vi "PupilAnalysis.vi"() -> ()   [LabVIEW 2013]
uses:
  <vilib>/picture/picture.llb/imagedata.ctl
  <vilib>/Analysis/baseanly.llb/Mean (DBL).vi
  <vilib>/Analysis/2dsp.llb/1D Convolution (DBL).vi
  <vilib>/Analysis/2dsp.llb/Decimate (single shot, DBL).vi
  <vilib>/Analysis/1siggen.llb/General Aperiodic Triangle.vi
  <vilib>/measure/maresamp.llb/Resample N Waveforms (single shot).vi
  <vilib>/measure/macond.llb/IIR Filter for N Chan.vi
  <vilib>/imath/engines/lvmath2/RunTimeEngine/ErrorHandling/NIMS_Finalize Error.vi
  <vilib>/imath/engines/lvmath2/RunTimeEngine/BuiltInFunctions/length/NIMS_length(GV).vi
  <instcachedir>/0/NIMS_length(GV)_08A3D13377FD4E4B96F5795FBF3698FA.lvgen/NIMS_length(GV)_08A3D13377FD4E4B96F5795FBF3698FA_000.vi
  <vilib>/imath/engines/lvmath2/RunTimeEngine/BuiltInFunctions/zeros/NIMS_V=zeros(I32,I32).vi
  <vilib>/imathl/engines/lvmath/Functions/Error Handling/Create Error.vi
  <vilib>/imath/engines/lvmath/Plug In/_Char/NIMS_CH_String to Character Array.vi
  <vilib>/imath/engines/lvmath2/RunTimeEngine/VariableToken/NIMS_VariableToken_CondDefined.vi
  <instcachedir>/0/NIMS_VariableToken_CondDefined_9DC5CEC47F8146B087FA2781C705B229.lvgen/NIMS_VariableToken_CondDefined_9DC5CEC47F8146B087FA2781C705B229_003.vi
  <vilib>/imath/engines/lvmath/Functions/Error Handling/MergeErrorsWrapper.vi
  <vilib>/imath/engines/lvmath2/RunTimeEngine/NodeEndStatement/NIMS_NodeEndStatement_Output.vi
  <instcachedir>/0/NIMS_NodeEndStatement_Output_53EC0D466D134D7ABD903AC30B43404B.lvgen/NIMS_NodeEndStatement_Output_53EC0D466D134D7ABD903AC30B43404B_005.vi
  <instcachedir>/0/NIMS_NodeEndStatement_Output_53EC0D466D134D7ABD903AC30B43404B.lvgen/NIMS_NodeEndStatement_Output_53EC0D466D134D7ABD903AC30B43404B_004.vi
  <vilib>/imath/engines/lvmath2/RunTimeEngine/RangeToken/NIMS_Range_R2 - Integer.vi
  <instcachedir>/0/NIMS_Range_R2 - Integer_C51C130E5EA5464EA148B28CDAB9615A.lvgen/NIMS_Range_R2 - Integer_C51C130E5EA5464EA148B28CDAB9615A_000.vi
  <vilib>/imath/engines/lvmath2/RunTimeEngine/CommandStatement/MC_CommandStatement_break.vi
  <vilib>/imath/engines/lvmath2/RunTimeEngine/IndexRead/NIMS V(S).vi
  <instcachedir>/0/NIMS V(S)_0488751826AF41519A22953C041130DC.lvgen/NIMS V(S)_0488751826AF41519A22953C041130DC_000.vi
  <vilib>/imath/engines/lvmath2/RunTimeEngine/ErrorHandling/NIMS_Create Error From Enums.vi
  <vilib>/imath/engines/lvmath2/RunTimeEngine/IndexReplace/NIMS V(S)=S.vi
  <instcachedir>/0/NIMS V(S)=S_66A18068148B4981A312229A93EA5C06.lvgen/NIMS V(S)=S_66A18068148B4981A312229A93EA5C06_003.vi
  <vilib>/imath/engines/lvmath2/RunTimeEngine/RangeToken/NIMS_Range.vi
  <instcachedir>/0/NIMS_Range_7481B155BEE341ECA0F59DDB444E2C09.lvgen/NIMS_Range_7481B155BEE341ECA0F59DDB444E2C09_000.vi
  <vilib>/imath/engines/lvmath2/RunTimeSupport/NIMS_Error if Not Equal.vi
  <instcachedir>/0/NIMS_Error if Not Equal_902F5D2649E64F5087A1EF57C55C58AB.lvgen/NIMS_Error if Not Equal_902F5D2649E64F5087A1EF57C55C58AB_001.vi
  <vilib>/imath/engines/lvmath2/RunTimeEngine/IndexRead/NIMS V(V).vi
  <instcachedir>/0/NIMS V(V)_298D9CB7BFEB42B8BC8D9C3C28AE8C70.lvgen/NIMS V(V)_298D9CB7BFEB42B8BC8D9C3C28AE8C70_000.vi
  <vilib>/imath/engines/lvmath2/RunTimeEngine/BuiltInFunctions/max/1 input/NIMS_max(RV).vi
  <instcachedir>/0/NIMS_max(RV)_237633DB1D604D5BA7001287DF3C7957.lvgen/NIMS_max(RV)_237633DB1D604D5BA7001287DF3C7957_002.vi
  <instcachedir>/0/NIMS V(S)_0488751826AF41519A22953C041130DC.lvgen/NIMS V(S)_0488751826AF41519A22953C041130DC_002.vi
  <vilib>/imath/engines/lvmath/Plug In/_Char/NIMS_CH_Character RV to String.vi
  <vilib>/imath/engines/lvmath2/RunTimeSupport/NIMS_String to Enum.vi
  <vilib>/imath/engines/lvmath2/RunTimeEngine/BuiltInFunctions/interpolate1d/NIMS_interpolate1d(RV,RV,RV,Str).vi
  <instcachedir>/0/NIMS_Error if Not Equal_902F5D2649E64F5087A1EF57C55C58AB.lvgen/NIMS_Error if Not Equal_902F5D2649E64F5087A1EF57C55C58AB_000.vi
  <instcachedir>/0/NIMS V(S)=S_66A18068148B4981A312229A93EA5C06.lvgen/NIMS V(S)=S_66A18068148B4981A312229A93EA5C06_000.vi
  <vilib>/imath/engines/lvmath2/RunTimeEngine/VariableToken/NIMS_VariableToken_CondDefinedDefinedByReplace.vi
  <instcachedir>/0/NIMS_VariableToken_CondDefinedDefinedByReplace_D162CFFC24174562A9FEA619A91E1A56.lvgen/NIMS_VariableToken_CondDefinedDefinedByReplace_D162CFFC24174562A9FEA619A91E1A56_002.vi
  <vilib>/Waveform/WDTFileIO.llb/ Write Waveforms to File (1D).vi
  <vilib>/Utility/file.llb/Read From Spreadsheet File (DBL).vi
  <vilib>/Utility/file.llb/Write To Spreadsheet File (DBL).vi
  <vilib>/Analysis/NI_AALBase.lvlib
  <vilib>/Analysis/NI_AALPro.lvlib
  <vilib>/measure/NI_MAPro.lvlib
  <vilib>/gmath/NI_Gmath.lvlib
panel:
  out "Tab Control":T1(tab)
  in  "Save Cleaned Data":bool
  in  "Apply New Settings":bool
  out "Cleaned Data":dynamicdata(graph)
  in  "New Sample Rate (Hz)":i32=25
  out "file information":string
  out "raw data":dbl[][](array[numeric])
  out "Unprocessed Data":waveform(dbl)[](graph)
  in  "Analyse Responses":bool
  in  "Rank":i32=3 min=1
  in  "Filter?":bool
  in  "Median Filter?":bool
  in  "max pupil width":dbl=0.4 format="%.2f"
  in  "min pupil width":dbl=0.1 format="%.2f"
  in  "min Aspect Ratio":dbl=0.7
  in  "Blink Window Length":dbl=5.0
  in  "Interpolation":u16(ring)=1 items=["Spline", "Linear"]
  in  "Resample Data":bool
  out "Sample Rate (Hz)":dbl format="%0.2f"
  in  "IIR filter specifications":T2={"Topology"=enum."Butterworth", "Type"=enum."Lowpass", "Order"=1, "Lower Fc"=10.0, "Upper Fc"=200.0, "PB Ripple"=1.0, "SB Attenuation"=60.0} {"PB Ripple" format="%0.2f"; "SB Attenuation" format="%0.2f"; "Lower Fc" format="%0.2p"; "Upper Fc" format="%0.2p"}
  out "Image onsets":string[](array[string])
  in  "Save Between Cursors":bool
  in  "Save Coefficients":bool
  out "Basis Set":dbl[][](graph)
  out "Event-related responses":dbl[][](graph)
  out "All Regressors":dbl[][](graph)
  out "Data and Fitted Response":dynamicdata(graph)
  in  "Timing Files":path[](array[path])
  in  "Number of Basis Functions":i32=15
  in  "Window Length (s)":dbl=10.0
  out "Coefficients":dbl[](array[numeric])
  in  "finished":bool
  in  "recalculate":bool
  in  "Save Response Data":bool
  in  "decimating factor":i32=1
  in  "Basis Set":u16(ring)=1 items=["Fourier", "Tents", "Blocks"]
  out "X * Y":dbl[](array[numeric])
  out "2D Picture":picture
  in  "next picture":bool
  out "image data":T3
  in  "Images Directory":path=path "E:/Documents/IAPS/bmp/800x600"
  in  "Objects Directory":path=path "E:/Documents/IAPS/objects"
  out "object file":path
  out "Image file":path
  out "Image Number":i32
  out "2D Picture 2":picture
  out "Fixations in ROIs":dbl[][](array[numeric])
  in  "Post-Picture Window Length":i32
  # "Data Cleaning"
  # "Pupil Dilation Analysis"
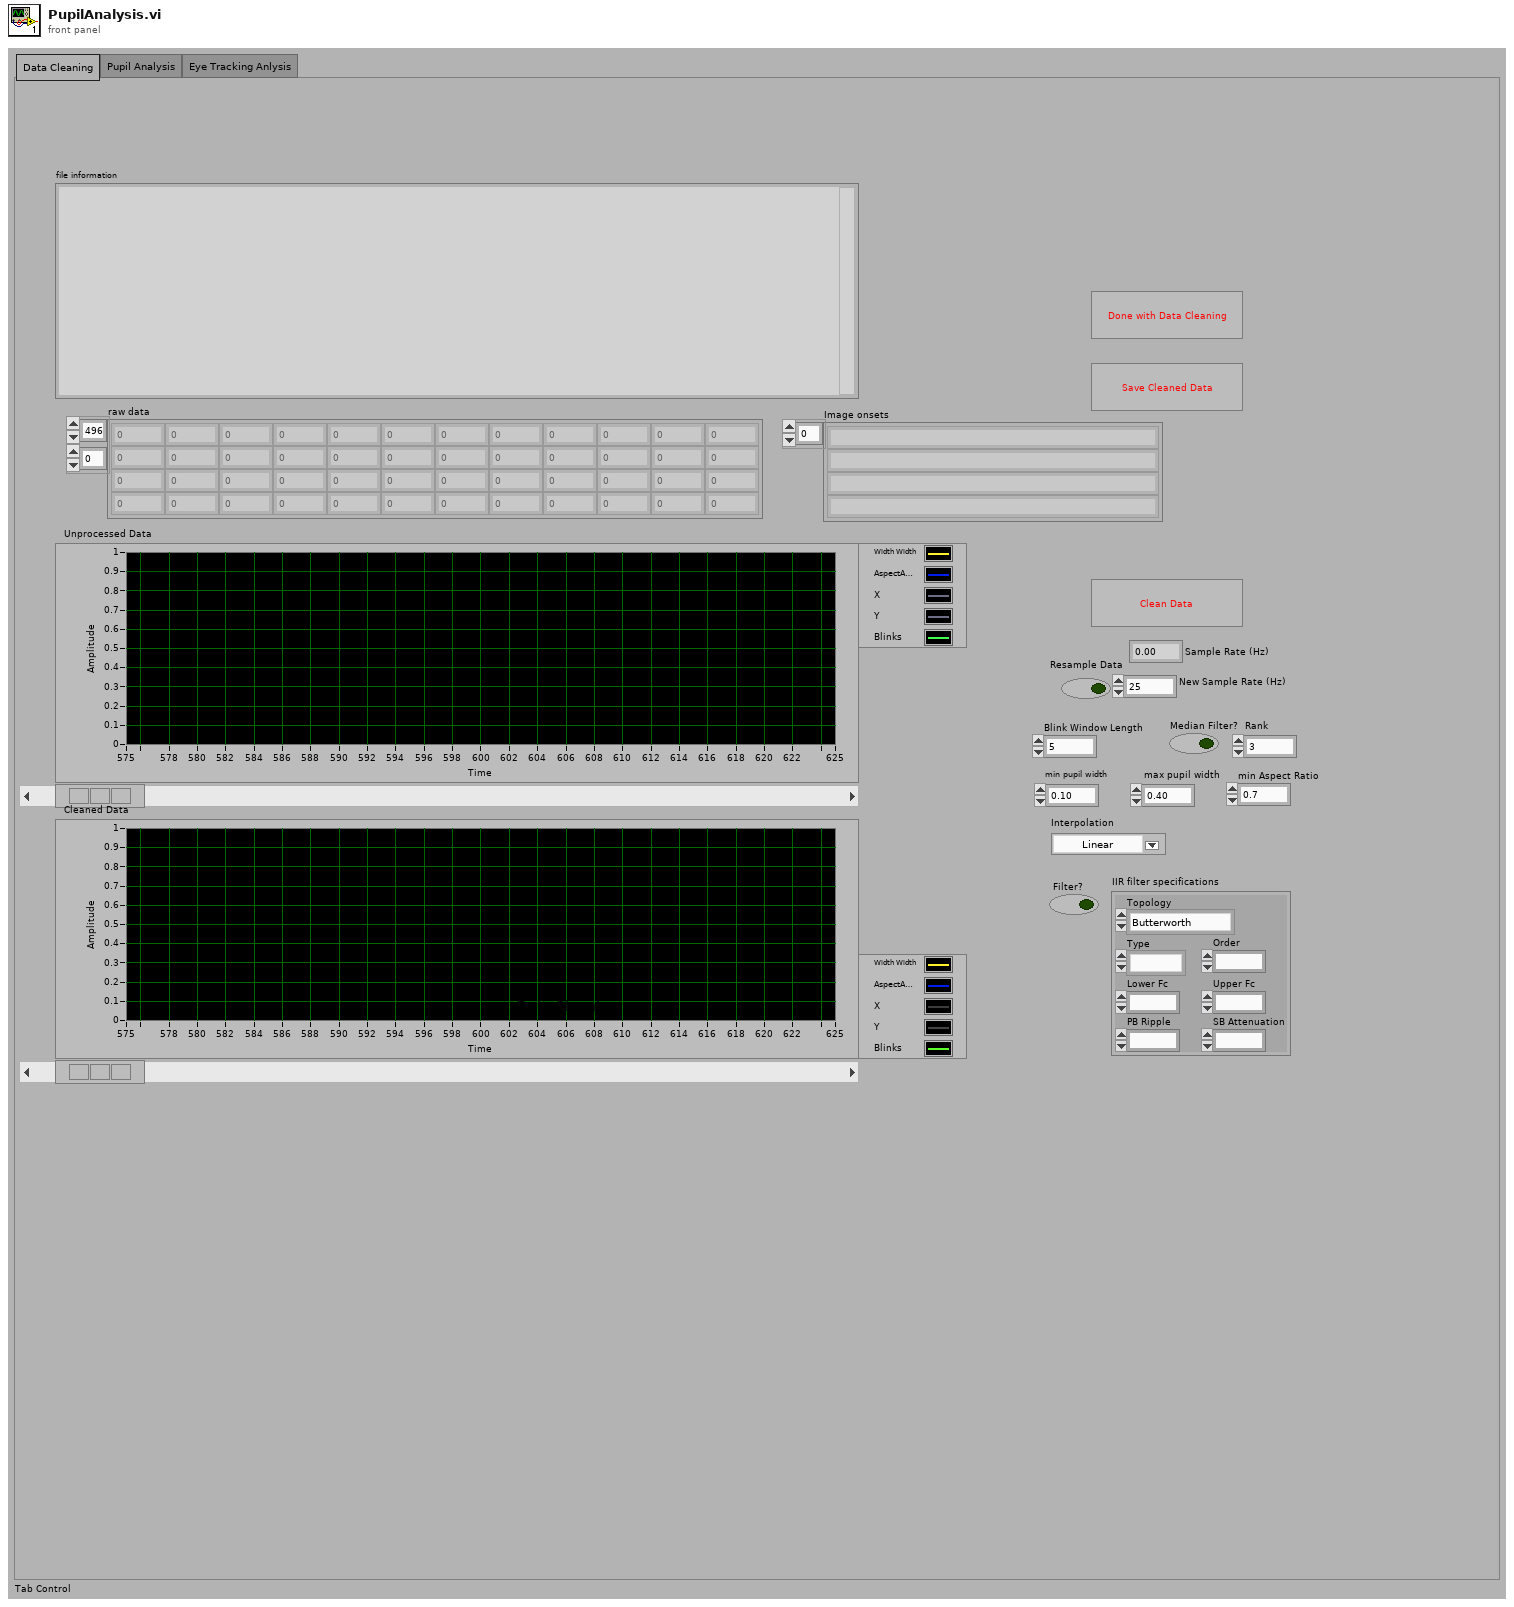
[diagram p1: front panel]
types:
  T1 = enum32{"Data Cleaning", "Pupil Analysis", "Eye Tracking Anlysis"}
  T2 = cluster{"Topology":enum16{"Off", "Butterworth", "Chebyshev", "Inverse Chebyshev", "Elliptic", "Bessel"}, "Type":enum16{"Lowpass", "Highpass", "Bandpass", "Bandstop"}, "Order":i32, "Lower Fc":dbl, "Upper Fc":dbl, "PB Ripple":dbl, "SB Attenuation":dbl}
  T3 = typedef "imagedata.ctl" = cluster{"image type":i32, "image depth":i32, "image":u8[], "mask":u8[], "colors":u32[], "Rectangle":cluster{"left":i16, "top":i16, "right":i16, "bottom":i16}}
  T4 = typedef "LVCursorListTypeDef.ctl" = cluster{"Name":string, "Color":u32, "Style":u8, "Point Style":u8, "Name Visible":bool, "Allow Drag":bool, "Cursor Mode":u32, "Plot":i32, "Index":i32, "Position":cluster{"X":dbl, "Y":dbl}, "X Scale":u32, "Y Scale":u32, "Watch Plots":i32[], "Watch All Plots":bool, "Plot Area":i32, "Label Offset":cluster{"X":dbl, "Y":dbl}}[]
  T5 = cluster{"Name":string, "Color":u32, "Style":u8, "Point Style":u8, "Name Visible":bool, "Allow Drag":bool, "Cursor Mode":u32, "Plot":i32, "Index":i32, "Position":cluster{"X":dbl, "Y":dbl}, "X Scale":u32, "Y Scale":u32, "Watch Plots":i32[], "Watch All Plots":bool, "Plot Area":i32, "Label Offset":cluster{"X":dbl, "Y":dbl}}
  T6 = cluster{"[0]":i32, "[1]":i32, "[2]":i32, "[3]":i32}
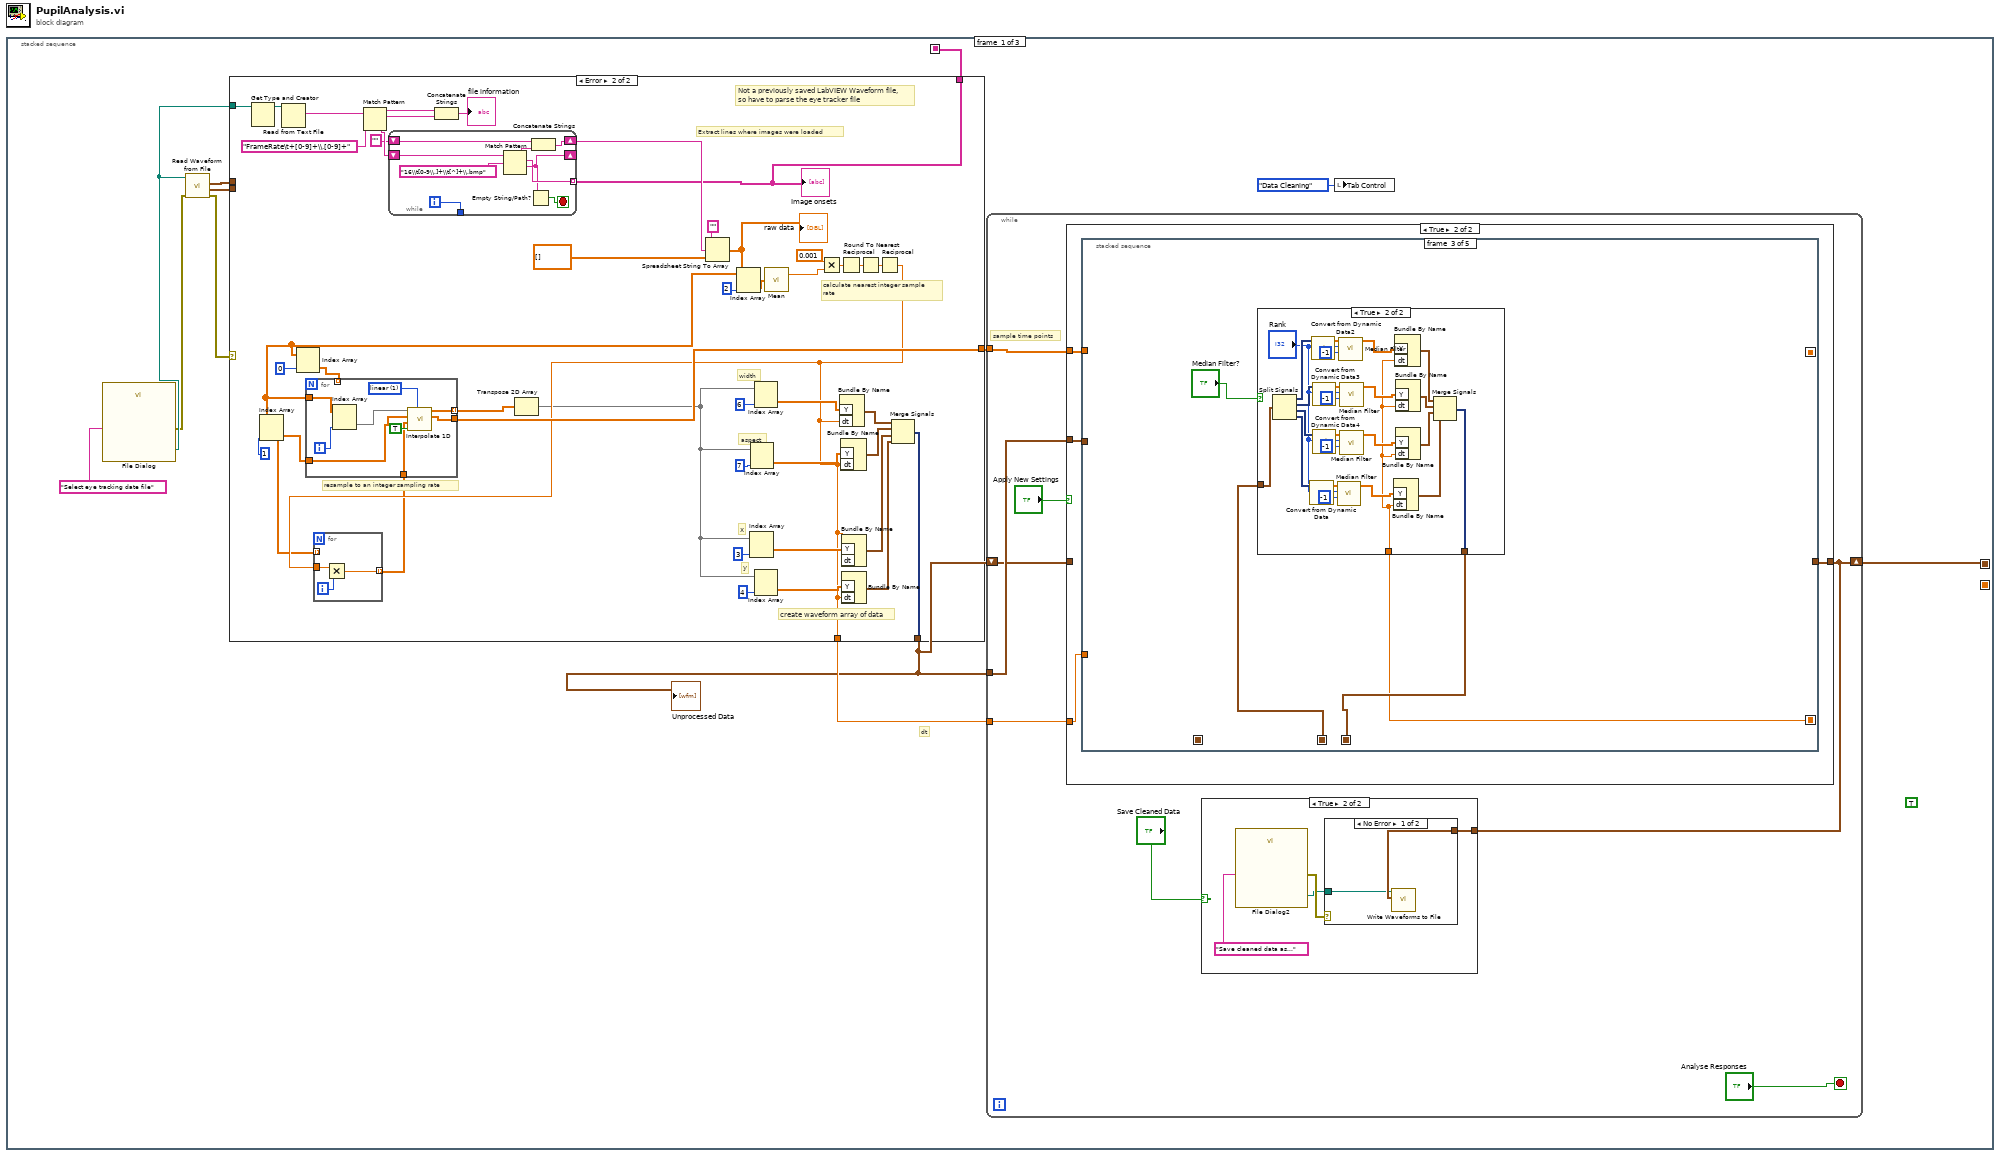
[diagram p0: block diagram]
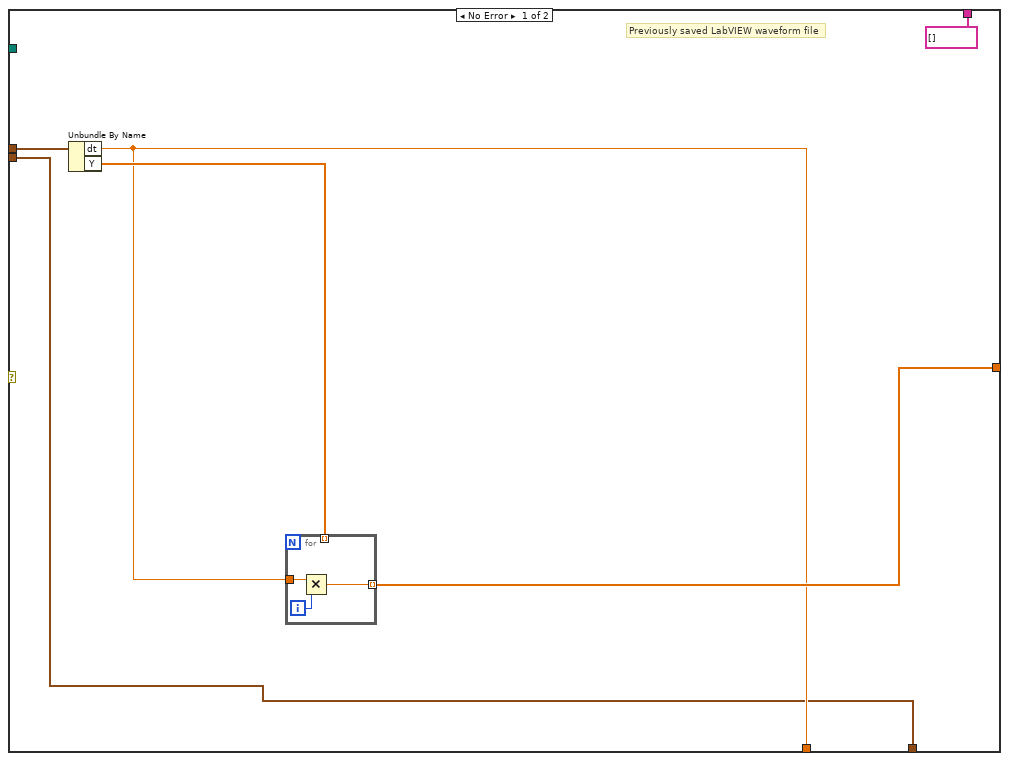
[diagram p2: hidden frame]
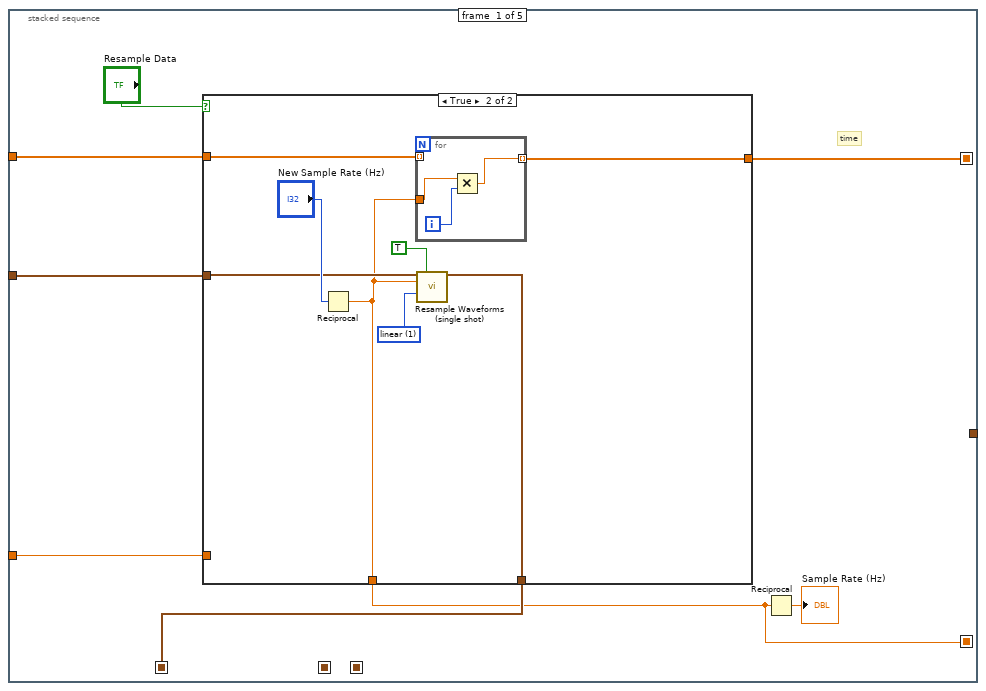
[diagram p6: hidden frame]
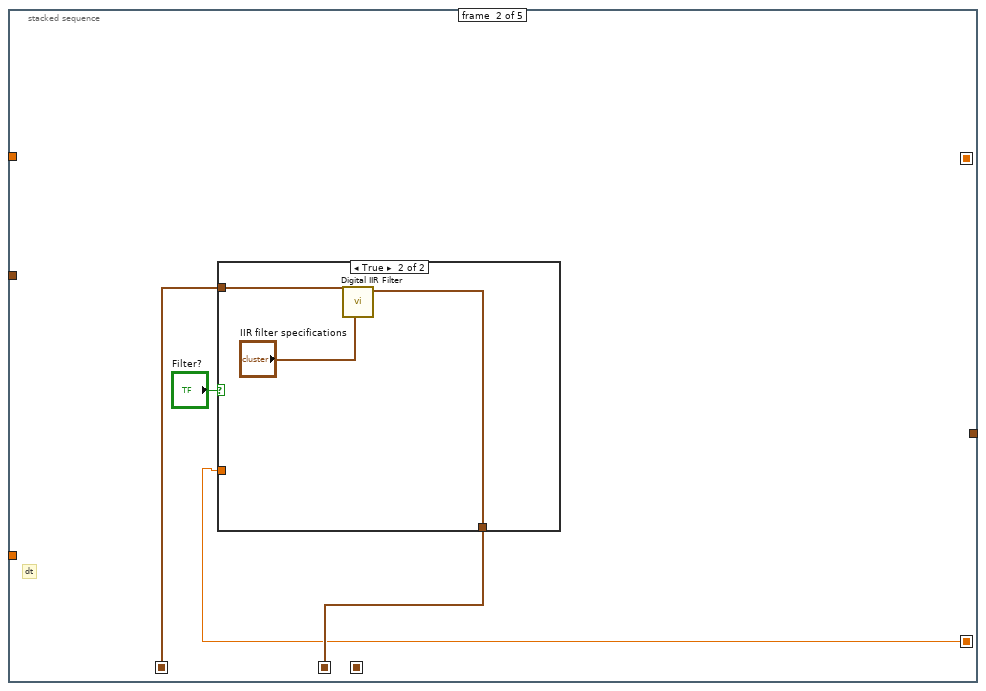
[diagram p8: hidden frame]
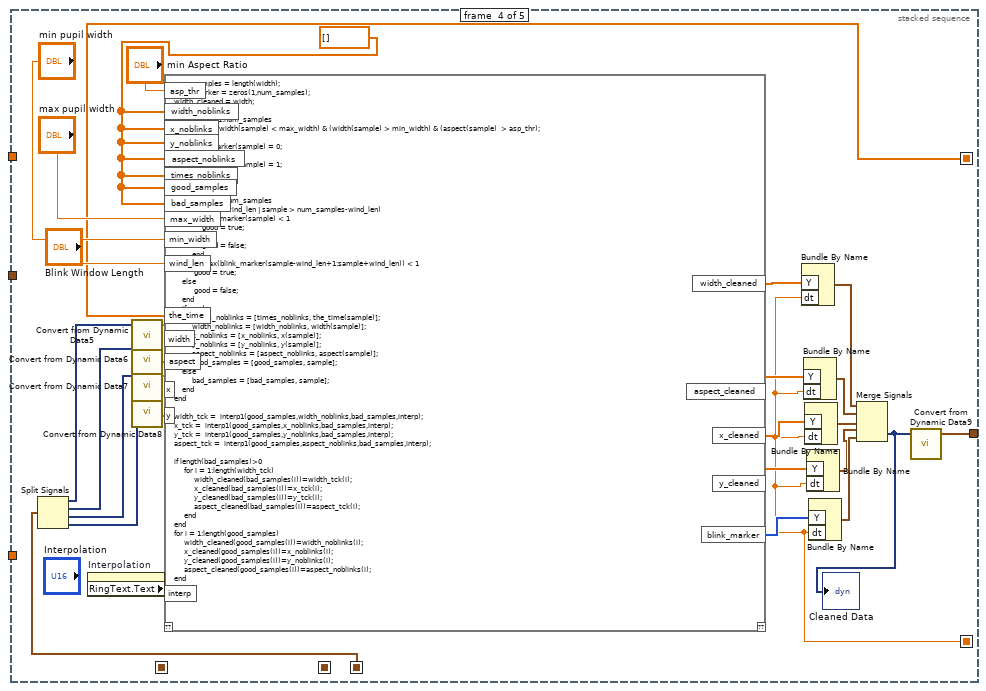
[diagram p11: hidden frame]
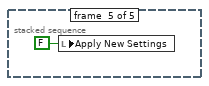
[diagram p12: hidden frame]
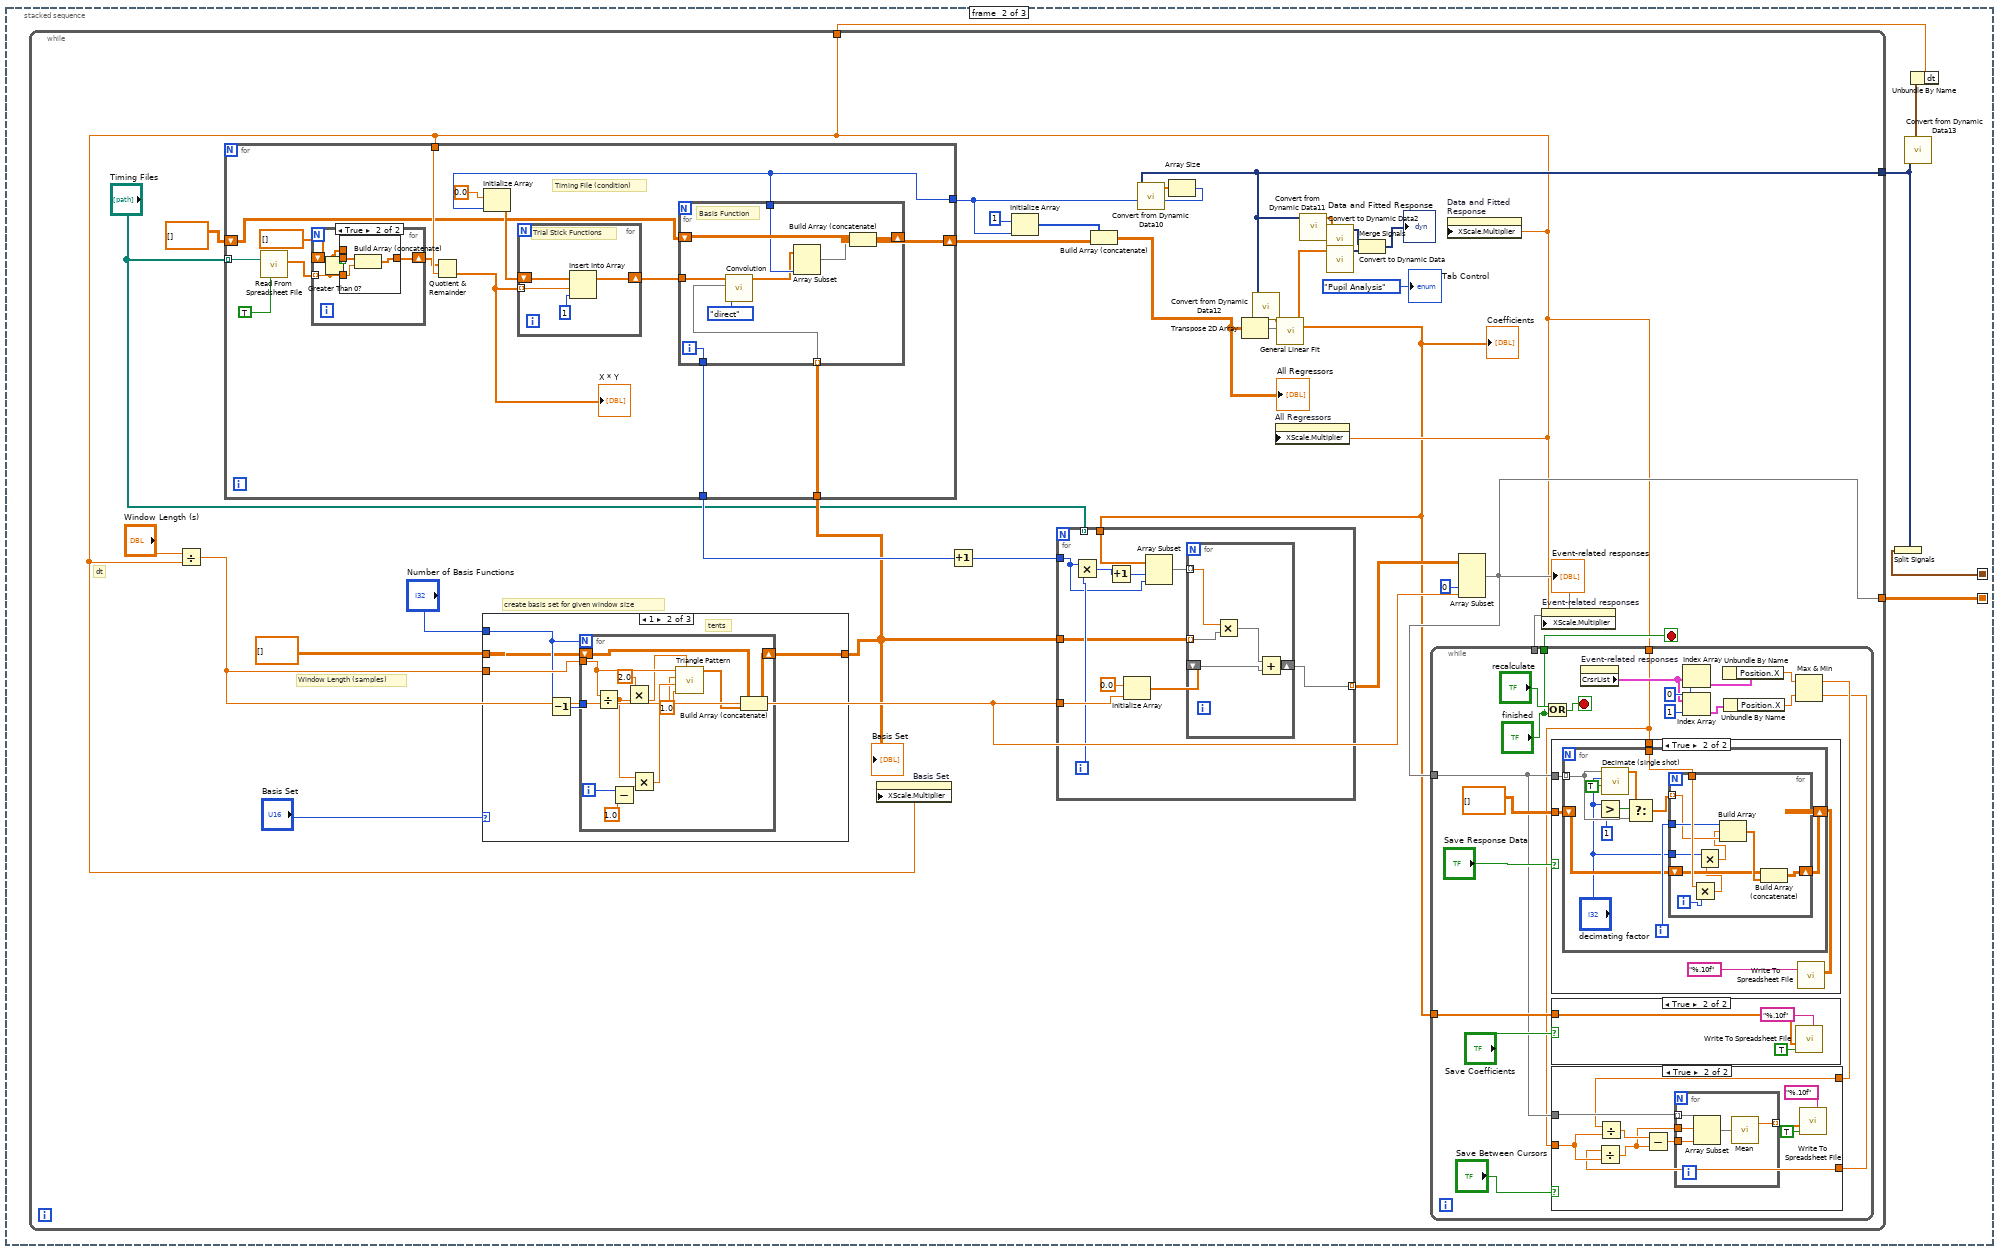
[diagram p13: hidden frame]
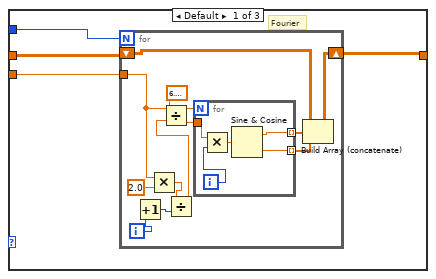
[diagram p14: hidden frame]
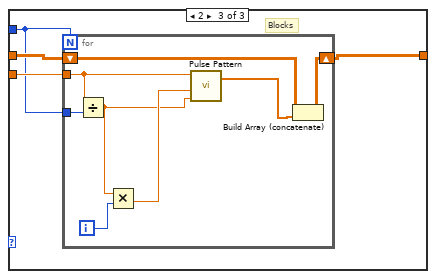
[diagram p15: hidden frame]
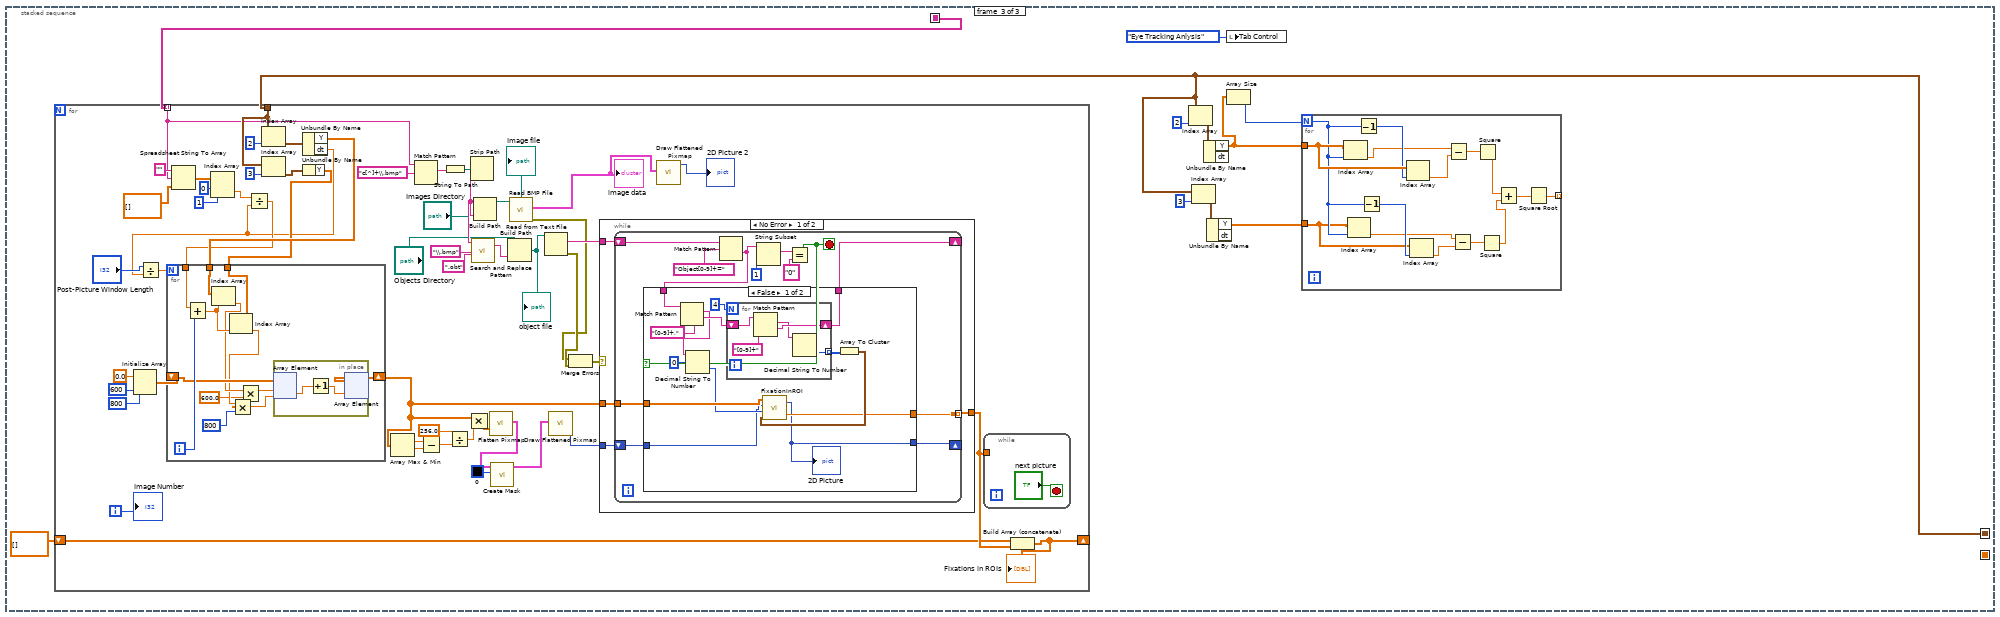
[diagram p20: hidden frame]
diagram:
  n1 = stacked-sequence {
    seq-local: [_ w1354 _] -> [_ _ _]
    seq-local: [w3 _ _] -> [_ w1353 w1554]
    seq-local: [w1 _ _] -> [_ _ w1555]
    frame #0 {
      (unwired) TRUE ("Median Filter?")
      # "dt"
      n2 = call "File Dialog"("prompt"="Select eye tracking date file") -> ("selected path"=w6:path, "error out"=w5:errorcluster)  [unwired: 11 in, 2 out]
      n3 = call <vilib>:"Read Waveform from File.vi"("error in (no error)"=w5, "file path (dialog if empty)"=w6) -> ("error out"=w7:errorcluster, "all waveforms in record"=w9:waveform(dbl)[], "first waveform in record"=w8:waveform(dbl))  [unwired: 4 in, 1 out]
      n4 = case shown="Error" w7 {
        tunnel: [w14 w45] -> w2
        tunnel: [w18 w37] -> w11
        tunnel: [w15 w36] -> w10
        tunnel: w6 -> [_ w27]
        tunnel: w9 -> [w14 _]
        tunnel: w8 -> [w17 _]
        tunnel: [string[] [] w23] -> w1
        frame No Error {
          # "Previously saved LabVIEW waveform file"
          n5 = Unbundle By Name(w17) -> ("dt"=w15:dbl, "Y"=w16:dbl[])
          n6 = for {
            tunnel: w15 -> [w20]
            tunnel: [w19] -> w18 mode=indexing
            tunnel: w16 -> [_] mode=indexing
            i -> [w21]
            n7 = Multiply(x=w20, y=w21) -> (x*y=w19:dbl)
          }
        }
        frame Error {
          # "Extract lines where images were loaded"
          # "create waveform array of data"
          # "resample to an integer sampling rate"
          # "calculate nearest integer sample\nrate"
          # "Not a previously saved LabVIEW Waveform file,\nso have to parse the eye tracker file"
          # "aspect"
          # "y"
          # "x"
          # "width"
          n8 = Get Type and Creator(7:w27) -> (3:w28:path)  [unwired: 1 in, 3 out]
          n9 = Read from Text File(file (use dialog)=w28) -> (text=w64:string)  [unwired: 3 in, 3 out]
          n10 = Match Pattern(string=w64, regular expression="FrameRate\t+[0-9]+\\.[0-9]+") -> (before substring=w62:string, match substring=w29:string, after substring=w26:string)  [unwired: 1 in, 1 out]
          n11 = while {
            shift-right: [w67] -> _
            shift-left: w26 -> [w73]
            shift-right: [w70] -> w25
            shift-left: "" -> [w72]
            tunnel: [w69] -> w23 mode=indexing
            tunnel: [w65] -> _
            i -> [w65]
            stop <- w68 stop-if-true
            n12 = Match Pattern(string=w73, regular expression="16\\t[0-9\\.]+\\t[^]+\\.bmp") -> (before substring=w71:string, match substring=w69:string, after substring=w67:string)  [unwired: 1 in, 1 out]
            n13 = Empty String/Path?(string/path=w67) -> (empty?=w68:bool)
            n14 = Concatenate Strings(w72, w71) -> (w70:string)
          }
          "Image onsets" <- w23
          n15 = Concatenate Strings(w62, w29) -> (→"file information":string)
          n16 = Spreadsheet String To Array(format string="", spreadsheet string=w25, array type (2D Dbl)=dbl[][] []) -> (array=w24:dbl[][])  [unwired: 1 in]
          "raw data" <- w24
          n17 = Index Array(array=w24, index (col)=1 ("disabled index (col)")) -> (element=w35:dbl[])  [unwired: 1 in]
          n18 = Index Array(array=w24, index (row)=0) -> (element=w32:dbl[])  [unwired: 1 in]
          n19 = Index Array(array=w24, index (col)=2) -> (element=w44:dbl[])  [unwired: 1 in]
          n20 = call-poly <vilib>:"Mean.vi"("X"=w44) -> ("mean"=w50:dbl)  [unwired: 1 out]
          n21 = Multiply(x=0.001, y=w50) -> (x*y=w41:dbl)
          n22 = Reciprocal(x=w41) -> (1/x=w38:dbl)
          n23 = Round To Nearest(number=w38) -> (nearest integer value=w39:dbl)
          n24 = Reciprocal(x=w39) -> (1/x=w36:dbl)
          n25 = for {
            tunnel: w36 -> [w75]
            tunnel: [w74] -> w34 mode=indexing
            tunnel: w35 -> [_] mode=indexing
            i -> [w76]
            n26 = Multiply(x=w75, y=w76) -> (x*y=w74:dbl)
          }
          n27 = for {
            tunnel: w24 -> [w81]
            tunnel: [w83] -> w40 mode=indexing
            tunnel: w35 -> [w78]
            tunnel: [w82] -> w37
            tunnel: w34 -> [w77]
            tunnel: w32 -> [_] mode=indexing
            i -> [w80]
            w84 = 1 items=["nearest", "linear", "spline", "cubic Hermite", "Lagrange"] ("method")
            n28 = Index Array(array=w81, index (col)=w80) -> (element=w79:dbl[])  [unwired: 1 in]
            n29 = call <vilib>:"Interpolate 1D.vi"("method"=w84, "X is monotonic"=TRUE, "xi"=w77, "X"=w78, "Y"=w79) -> ("xi used"=w82:dbl[], "yi"=w83:dbl[])  [unwired: 4 in, 1 out]
          }
          n30 = Transpose 2D Array(2D array=w40) -> (transposed array=w31:dbl[][])
          n31 = Index Array(array=w31, index (col)=3 ("disabled index (col)")) -> (element=w53:dbl[])  [unwired: 1 in]
          n32 = Index Array(array=w31, index (col)=7 ("disabled index (col)")) -> (element=w51:dbl[])  [unwired: 1 in]
          n33 = Index Array(array=w31, index (col)=6 ("disabled index (col)")) -> (element=w54:dbl[])  [unwired: 1 in]
          n34 = Index Array(array=w31, index (col)=4 ("disabled index (col)")) -> (element=w52:dbl[])  [unwired: 1 in]
          n35 = Bundle By Name("Y"=w54, "dt"=w36) -> (w49:waveform(dbl))  [unwired: 1 in]
          n36 = Bundle By Name("Y"=w51, "dt"=w36) -> (w48:waveform(dbl))  [unwired: 1 in]
          n37 = Bundle By Name("Y"=w53, "dt"=w36) -> (w47:waveform(dbl))  [unwired: 1 in]
          n38 = Bundle By Name("Y"=w52, "dt"=w36) -> (w46:waveform(dbl))  [unwired: 1 in]
          n39 = Merge Signals(w49, w48, w47, w46) -> (w45:dynamicdata)
        }
      }
      "Unprocessed Data" <- w2
      n40 = while {
        tunnel: w10 -> [w91]
        tunnel: w2 -> [w92]
        tunnel: w11 -> [w93]
        shift-right: [w87] -> w3
        shift-left: w2 -> [w86]
        stop <- "Analyse Responses" stop-if-true
        # "sample time points"
        n41 = case shown="True" "Apply New Settings" {
          tunnel: w93 -> [_ w104]
          tunnel: w92 -> [_ w103]
          tunnel: w91 -> [_ w102]
          tunnel: [w100 w101] -> w87
          tunnel: w86 -> [w100 _]
          frame False {
          }
          frame True {
            n42 = stacked-sequence {
              seq-local: [_ w130 _ _ _] -> [_ _ w138 _ _]
              seq-local: [_ _ w136 _ _] -> [_ _ _ w185 _]
              seq-local: [w111 _ _ _ _] -> [_ w128 _ _ _]
              seq-local: [w109 _ _ _ _] -> [_ _ _ w176 _]
              seq-local: [w106 _ _ _ _] -> [_ w127 w135 w167 _]
              tunnel: w104 -> [w110 _ _ _ _]
              tunnel: w102 -> [w105 _ _ _ _]
              tunnel: w103 -> [w108 _ _ _ _]
              tunnel: [_ _ _ w165 _] -> w101
              frame #0 {
                # "time"
                n43 = case shown="True" "Resample Data" {
                  tunnel: [w115 w118] -> w111
                  tunnel: w108 -> [w115 w120]
                  tunnel: w110 -> [w114 w123]
                  tunnel: [w114 w121] -> w109
                  tunnel: [w113 w117] -> w106
                  tunnel: w105 -> [w113 _]
                  frame False {
                  }
                  frame True {
                    w119 = u16 1 items=["coerce", "linear", "spline", "FIR filter"] ("interpolation mode")
                    n44 = Reciprocal(x="New Sample Rate (Hz)") -> (1/x=w117:dbl)
                    n45 = for {
                      tunnel: w123 -> [_] mode=indexing
                      tunnel: w117 -> [w126]
                      tunnel: [w124] -> w121 mode=indexing
                      i -> [w125]
                      n46 = Multiply(x=w126, y=w125) -> (x*y=w124:dbl)
                    }
                    n47 = call-poly <vilib>:"Resample Waveforms (single shot).vi"("waveforms in"=w120, "open interval? (F)"=TRUE, "dt"=w117, "interpolation mode"=w119) -> ("resampled waveforms out"=w118:waveform(dbl)[])  [unwired: 8 in, 3 out]
                  }
                }
                n48 = Reciprocal(x=w106) -> (1/x=→"Sample Rate (Hz)":dbl)
              }
              frame #1 {
                # "dt"
                n49 = case shown="True" "Filter?" {
                  tunnel: w128 -> [w131 w134]
                  tunnel: [w131 w132] -> w130
                  tunnel: w127 -> [_ _]
                  frame False {
                  }
                  frame True {
                    n50 = call-poly <vilib>:"Digital IIR Filter.vi"("IIR filter specifications"="IIR filter specifications", "signal(s) in"=w134) -> ("signal(s) out"=w132:waveform(dbl)[])  [unwired: 7 in, 2 out]
                  }
                }
              }
              frame #2 {
                n51 = case shown="True" "Median Filter?" {
                  tunnel: w138 -> [w139 w161]
                  tunnel: [w139 w142] -> w136
                  tunnel: w135 -> [_ w141]
                  frame False {
                  }
                  frame True {
                    n52 = Split Signals(w161) -> (w147:dynamicdata, w148:dynamicdata, w149:dynamicdata, w160:dynamicdata)  [unwired: 4 in]
                    n53 = call "Convert from Dynamic Data"("Dynamic Data Type"=w160) -> ("Array"=w159:dbl[])  [unwired: 3 in]
                    n54 = call "Convert from Dynamic Data2"("Dynamic Data Type"=w147) -> ("Array"=w156:dbl[])  [unwired: 3 in]
                    n55 = call "Convert from Dynamic Data3"("Dynamic Data Type"=w148) -> ("Array"=w153:dbl[])  [unwired: 3 in]
                    n56 = call "Convert from Dynamic Data4"("Dynamic Data Type"=w149) -> ("Array"=w150:dbl[])  [unwired: 3 in]
                    n57 = call <vilib>:"Median Filter.vi"("right rank"=-1, "left rank"="Rank", "X"=w159) -> ("Filtered X"=w162:dbl[])  [unwired: 7 in, 1 out]
                    n58 = call <vilib>:"Median Filter.vi"("right rank"=-1, "left rank"="Rank", "X"=w156) -> ("Filtered X"=w157:dbl[])  [unwired: 7 in, 1 out]
                    n59 = call <vilib>:"Median Filter.vi"("right rank"=-1, "left rank"="Rank", "X"=w153) -> ("Filtered X"=w154:dbl[])  [unwired: 7 in, 1 out]
                    n60 = call <vilib>:"Median Filter.vi"("right rank"=-1, "left rank"="Rank", "X"=w150) -> ("Filtered X"=w151:dbl[])  [unwired: 7 in, 1 out]
                    n61 = Bundle By Name("Y"=w162, "dt"=w141) -> (w143:waveform(dbl))  [unwired: 1 in]
                    n62 = Bundle By Name("Y"=w157, "dt"=w141) -> (w146:waveform(dbl))  [unwired: 1 in]
                    n63 = Bundle By Name("Y"=w154, "dt"=w141) -> (w145:waveform(dbl))  [unwired: 1 in]
                    n64 = Bundle By Name("Y"=w151, "dt"=w141) -> (w144:waveform(dbl))  [unwired: 1 in]
                    n65 = Merge Signals(w146, w145, w144, w143) -> (w142:dynamicdata)
                  }
                }
              }
              frame #3 {
                w164 = dbl[] []
                n66 = Split Signals(w185) -> (w184:dynamicdata, w182:dynamicdata, w180:dynamicdata, w178:dynamicdata)  [unwired: 4 in]
                n67 = property on="Interpolation" class="Ring (strict)"() -> ("RingText.Text"=w187:string)  [unwired: 2 in, 2 out]
                n68 = call "Convert from Dynamic Data5"("Dynamic Data Type"=w184) -> ("Array"=w183:dbl[])  [unwired: 3 in]
                n69 = call "Convert from Dynamic Data6"("Dynamic Data Type"=w182) -> ("Array"=w181:dbl[])  [unwired: 3 in]
                n70 = call "Convert from Dynamic Data7"("Dynamic Data Type"=w180) -> ("Array"=w179:dbl[])  [unwired: 3 in]
                n71 = call "Convert from Dynamic Data8"("Dynamic Data Type"=w178) -> ("Array"=w177:dbl[])  [unwired: 3 in]
                n72 = mathscript code="num_samples = length(width);\nblink_marker = zeros(1,num_samples);\nwidth_cleaned = width;\n\nfor sample =1:num_samples\n    noblink = (width(sample) < max_width) & (width(sample) > min_width) & (aspect(sample)  > asp_thr);\n    if noblink\n\t      \tblink_marker(sample) = 0;\n    else\n\t      \tblink_marker(sample) = 1;\n    end\nend\n\nfor sample =1:num_samples\n    if (sample < wind_len | sample > num_samples-wind_len)\n         if  blink_marker(sample) < 1\n              good = true;\n         else\n              good = false;\n         end\n    elseif max(blink_marker(sample-wind_len+1:sample+wind_len)) < 1\n\t         good = true;\n    else\n          good = false;\n    end\n    if good\n        \ttimes_noblinks = [times_noblinks, the_time(sample)];\n\t\t      \twidth_noblinks = [width_noblinks, width(sample)];\n\t\t      \tx_noblinks = [x_noblinks, x(sample)];\n\t\t\t      y_noblinks = [y_noblinks, y(sample)];\n         aspect_noblinks = [aspect_noblinks, aspect(sample)];\n\t\t  \t    good_samples = [good_samples, sample];\n    else\n         bad_samples = [bad_samples, sample];\n    end\nend\n\nwidth_tck =  interp1(good_samples,width_noblinks,bad_samples,interp);\nx_tck =  interp1(good_samples,x_noblinks,bad_samples,interp);\ny_tck =  interp1(good_samples,y_noblinks,bad_samples,interp);\naspect_tck =  interp1(good_samples,aspect_noblinks,bad_samples,interp);\n\nif length(bad_samples)>0\n     for i = 1:length(width_tck)\n          width_cleaned(bad_samples(i))=width_tck(i);\n          x_cleaned(bad_samples(i))=x_tck(i);\n          y_cleaned(bad_samples(i))=y_tck(i);\n          aspect_cleaned(bad_samples(i))=aspect_tck(i);\n     end\nend\nfor i = 1:length(good_samples)\n     width_cleaned(good_samples(i))=width_noblinks(i);\n     x_cleaned(good_samples(i))=x_noblinks(i);\n     y_cleaned(good_samples(i))=y_noblinks(i);\n     aspect_cleaned(good_samples(i))=aspect_noblinks(i);\nend"("width"=w183, "aspect"=w181, "asp_thr"="min Aspect Ratio", "min_width"="min pupil width", "wind_len"="Blink Window Length", "x"=w179, "y"=w177, "the_time"=w176, "max_width"="max pupil width", "interp"=w187, "width_noblinks"=w164, "x_noblinks"=w164, "y_noblinks"=w164, "aspect_noblinks"=w164, "times_noblinks"=w164, "good_samples"=w164, "bad_samples"=w164) -> ("blink_marker"=w191:i32[], "width_cleaned"=w186:dbl[], "aspect_cleaned"=w175:dbl[], "x_cleaned"=w174:dbl[], "y_cleaned"=w173:dbl[])  [unwired: 1 in, 1 out]
                n73 = Bundle By Name("Y"=w186, "dt"=w167) -> (w172:waveform(dbl))  [unwired: 1 in]
                n74 = Bundle By Name("Y"=w175, "dt"=w167) -> (w171:waveform(dbl))  [unwired: 1 in]
                n75 = Bundle By Name("Y"=w174, "dt"=w167) -> (w170:waveform(dbl))  [unwired: 1 in]
                n76 = Bundle By Name("Y"=w173, "dt"=w167) -> (w168:waveform(dbl))  [unwired: 1 in]
                n77 = Bundle By Name("Y"=w191, "dt"=w167) -> (w169:waveform(i32))  [unwired: 1 in]
                n78 = Merge Signals(w172, w171, w170, w168, w169) -> (w166:dynamicdata)
                "Cleaned Data" <- w166
                n79 = call "Convert from Dynamic Data9"("Dynamic Data Type"=w166) -> ("Array of Waveform"=w165:waveform(dbl)[])  [unwired: 3 in]
              }
              frame #4 {
                n80 = local write "Apply New Settings"(FALSE ("Apply New Settings")) -> ()
              }
            }
          }
        }
        n81 = case shown="True" "Save Cleaned Data" {
          tunnel: w87 -> [_ w95]
          frame False {
          }
          frame True {
            n82 = call "File Dialog2"("prompt"="Save cleaned data as...") -> ("selected path"=w94:path, "error out"=w96:errorcluster)  [unwired: 11 in, 2 out]
            n83 = case shown="No Error" w96 {
              tunnel: w95 -> [w99 _]
              tunnel: w94 -> [w98 _]
              frame No Error {
                n84 = call-poly <vilib>:"Write Waveforms to File.vi"("waveform array"=w99, "file path (dialog if empty)"=w98) -> ()  [unwired: 8 in, 2 out]
              }
              frame Error {
              }
            }
          }
        }
      }
      n85 = local write "Tab Control"(enum32{"Data Cleaning", "Pupil Analysis"}."Data Cleaning" ("Tab Control")) -> ()
    }
    frame #1 {
      n86 = Split Signals(w1353) -> (w1352:dynamicdata)  [unwired: 1 in]
      n87 = call "Convert from Dynamic Data13"("Dynamic Data Type"=w1352) -> ("Waveform"=w1351:waveform(dbl))  [unwired: 3 in]
      n88 = Unbundle By Name(w1351) -> ("dt"=w1350:dbl)
      n89 = while {
        tunnel: w1352 -> [w1382]
        tunnel: w1350 -> [w1366]
        tunnel: [w1369] -> w1354
        stop <- w1370 stop-if-true
        # "create basis set for given window size"
        # "dt"
        # "Window Length (samples)"
        n90 = Divide(x="Window Length (s)", y=w1366) -> (x/y=w1367:dbl)
        n91 = case shown="1" "Basis Set" {
          tunnel: w1367 -> [w1389 w1411 w1428]
          tunnel: "Number of Basis Functions" -> [w1386 w1408 w1425]
          tunnel: [w1388 w1410 w1427] -> w1363
          tunnel: dbl[][] [] -> [w1387 w1407 w1426]
          frame Default {
            # "Fourier"
            n92 = for {
              N: w1386 -> [_]
              tunnel: w1389 -> [w1397]
              shift-right: [w1392] -> w1388
              shift-left: w1387 -> [w1391]
              i -> [w1390]
              n93 = Increment(x=w1390) -> (x+1=w1393:i32)
              n94 = Multiply(x=w1397, y=2.0) -> (x*y=w1395:dbl)
              n95 = Divide(x=w1395, y=w1393) -> (x/y=w1394:dbl)
              n96 = Divide(x=6.283185307179586, y=w1394) -> (x/y=w1400:dbl)
              n97 = for {
                N: w1397 -> [_]
                tunnel: [w1406] -> w1399 mode=indexing
                tunnel: [w1405] -> w1398 mode=indexing
                tunnel: w1400 -> [w1402]
                i -> [w1403]
                n98 = Multiply(x=w1402, y=w1403) -> (x*y=w1404:dbl)
                n99 = Sine & Cosine(0:w1404) -> (1:w1406:dbl, 2:w1405:dbl)
              }
              n100 = Build Array (concatenate)(w1391, w1399, w1398) -> (w1392:dbl[][])
            }
          }
          frame 1 {
            # "tents"
            n101 = Decrement(x=w1408) -> (x-1=w1409:i32)
            n102 = for {
              N: w1408 -> [_]
              tunnel: w1409 -> [w1424]
              tunnel: w1411 -> [w1423]
              shift-right: [w1415] -> w1410
              shift-left: w1407 -> [w1416]
              i -> [w1414]
              w1412 = 1.0 ("delta t (s)")
              n103 = Divide(x=w1423, y=w1424) -> (x/y=w1417:dbl)
              n104 = Subtract(x=w1414, y=1.0) -> (x-y=w1420:dbl)
              n105 = Multiply(x=2.0, y=w1417) -> (x*y=w1418:dbl)
              n106 = Multiply(x=w1417, y=w1420) -> (x*y=w1421:dbl)
              n107 = call <vilib>:"Triangle Pattern.vi"("width (s)"=w1418, "delta t (s)"=w1412, "delay (s)"=w1421, "amplitude"=w1412, "samples"=w1423) -> ("Triangle Pattern"=w1413:dbl[])  [unwired: 5 in, 1 out]
              n108 = Build Array (concatenate)(w1416, w1413) -> (w1415:dbl[][])
            }
          }
          frame 2 {
            # "Blocks"
            n109 = for {
              N: w1425 -> [_]
              tunnel: w1425 -> [w1436]
              tunnel: w1428 -> [w1430]
              shift-right: [w1434] -> w1427
              shift-left: w1426 -> [w1433]
              i -> [w1435]
              n110 = Divide(x=w1430, y=w1436) -> (x/y=w1431:dbl)
              n111 = Multiply(x=w1431, y=w1435) -> (x*y=w1432:dbl)
              n112 = call <vilib>:"Pulse Pattern.vi"("width"=w1431, "delay"=w1432, "samples"=w1430) -> ("Pulse Pattern"=w1429:dbl[])  [unwired: 1 in, 1 out]
              n113 = Build Array (concatenate)(w1433, w1429) -> (w1434:dbl[][])
            }
          }
        }
        "Basis Set" <- w1363
        n114 = property on="Basis Set" class="WFGraph (strict)"("XScale.Multiplier"=w1366) -> ()  [unwired: 2 in, 2 out]
        n115 = call "Convert from Dynamic Data10"("Dynamic Data Type"=w1382) -> ("Array"=w1358:dbl[])  [unwired: 3 in]
        n116 = Array Size(array=w1358) -> (size(s)=w1377:i32)
        n117 = for {
          tunnel: "Timing Files" -> [w1530] mode=indexing
          shift-right: [w1522] -> w1362
          shift-left: dbl[][] [] -> [w1523]
          tunnel: w1377 -> [w1521]
          tunnel: w1366 -> [w1528]
          tunnel: w1363 -> [w1525]
          tunnel: [w1524] -> w1374
          # "Timing File (condition)"
          n118 = call-poly <vilib>:"Read From Spreadsheet File.vi"("transpose (no:F)"=TRUE, "file path (dialog if empty)"=w1530) -> ("first row"=w1518:dbl[])  [unwired: 5 in, 4 out]
          n119 = for {
            shift-right: [w1534] -> w1517
            shift-left: dbl[] [] -> [w1531]
            tunnel: w1518 -> [w1533] mode=indexing
            n120 = Greater Than 0?(x=w1533) -> (x > 0?=w1532:bool)
            n121 = case shown="True" w1532 {
              tunnel: w1531 -> [_ w1538]
              tunnel: w1533 -> [_ w1537]
              tunnel: [w1535 w1536] -> w1534
              tunnel: w1531 -> [w1535 _]
              frame False {
              }
              frame True {
                n122 = Build Array (concatenate)(w1538, w1537) -> (w1536:dbl[])
              }
            }
          }
          n123 = Quotient & Remainder(x=w1517, y=w1528) -> (floor(x/y)=w1519:dbl[])  [unwired: 1 out]
          "X * Y" <- w1519
          n124 = Initialize Array(0.0 ("element"), w1521) -> (w1526:dbl[])
          n125 = for {
            shift-right: [w1540] -> w1520
            shift-left: w1526 -> [w1542]
            tunnel: w1519 -> [w1539] mode=indexing
            # "Trial Stick Functions"
            n126 = Insert Into Array(array=w1542, index=w1539, new element=1) -> (w1540:dbl[])
          }
          n127 = for {
            tunnel: w1525 -> [w1544] mode=indexing
            tunnel: w1520 -> [w1543]
            tunnel: [w1551] -> w1524
            shift-right: [w1550] -> w1522
            shift-left: w1523 -> [w1549]
            tunnel: w1521 -> [w1548]
            i -> [w1551]
            # "Basis Function"
            n128 = call-poly <vilib>:"Convolution.vi"("algorithm"=enum32{"direct", "frequency domain"}."direct", "Y"=w1544, "X"=w1543) -> ("X * Y"=w1545:dbl[])  [unwired: 7 in, 1 out]
            n129 = Array Subset(array=w1545, length=w1548) -> (w1547:dbl[])  [unwired: 1 in]
            n130 = Build Array (concatenate)(w1549, w1547) -> (w1550:dbl[][])
          }
        }
        n131 = Increment(x=w1374) -> (x+1=w1360:i32)
        n132 = Initialize Array(1 ("element"), w1377) -> (w1361:i32[])
        n133 = Build Array (concatenate)(w1361, w1362) -> (w1371:dbl[][])
        "All Regressors" <- w1371
        n134 = Transpose 2D Array(2D array=w1371) -> (transposed array=w1379:dbl[][])
        n135 = call "Convert from Dynamic Data12"("Dynamic Data Type"=w1382) -> ("Array"=w1356:dbl[])  [unwired: 3 in]
        n136 = property on="All Regressors" class="WFGraph (strict)"("XScale.Multiplier"=w1366) -> ()  [unwired: 2 in, 2 out]
        n137 = call <vilib>:"General Linear Fit.vi"("Y"=w1356, "H"=w1379) -> ("Best Fit"=w1384:dbl[], "Coefficients"=w1355:dbl[])  [unwired: 8 in, 4 out]
        "Coefficients" <- w1355
        n138 = for {
          tunnel: w1355 -> [w1510]
          tunnel: "Timing Files" -> [_] mode=indexing
          tunnel: [w1502] -> w1375 mode=indexing
          tunnel: w1367 -> [w1508]
          tunnel: w1360 -> [w1501]
          tunnel: w1363 -> [w1503]
          i -> [w1505]
          n139 = Multiply(x=w1501, y=w1505) -> (x*y=w1504:i32)
          n140 = Increment(x=w1504) -> (x+1=w1500:i32)
          n141 = Initialize Array(0.0 ("element"), w1508) -> (w1506:dbl[])
          n142 = Array Subset(array=w1510, index=w1500, length=w1501) -> (w1509:dbl[])
          n143 = for {
            tunnel: w1509 -> [w1515] mode=indexing
            shift-right: [w1511] -> w1502
            shift-left: w1506 -> [w1512]
            tunnel: w1503 -> [w1514] mode=indexing
            n144 = Multiply(x=w1515, y=w1514) -> (x*y=w1513:dbl[])
            n145 = Add(x=w1513, y=w1512) -> (x+y=w1511:dbl[])
          }
        }
        n146 = call "Convert from Dynamic Data11"("Dynamic Data Type"=w1382) -> ("Array"=w1357:dbl[])  [unwired: 3 in]
        n147 = call "Convert to Dynamic Data2"("Array"=w1357) -> ("Dynamic Data Type"=w1381:dynamicdata)  [unwired: 3 in]
        n148 = call "Convert to Dynamic Data"("Array"=w1384) -> ("Dynamic Data Type"=w1383:dynamicdata)  [unwired: 3 in]
        n149 = Merge Signals(w1381, w1383) -> (→"Data and Fitted Response":dynamicdata)
        n150 = property on="Data and Fitted Response" class="WFGraph (strict)"("XScale.Multiplier"=w1366) -> ()  [unwired: 2 in, 2 out]
        n151 = Array Subset(array=w1375, index (col)=0 ("index"), length (col)=w1367) -> (w1369:dbl[][])  [unwired: 2 in]
        "Event-related responses" <- w1369
        n152 = while {
          tunnel: w1369 -> [_]
          tunnel: ["finished"] -> w1370
          tunnel: w1369 -> [w1447]
          tunnel: w1366 -> [w1437]
          tunnel: w1355 -> [w1451]
          stop <- w1454 stop-if-true
          n153 = Or(x="recalculate", y="finished") -> (x .or. y?=w1454:bool)
          n154 = case shown="True" "Save Response Data" {
            tunnel: w1447 -> [_ w1478]
            tunnel: w1437 -> [_ w1477]
            tunnel: dbl[][] [] -> [_ w1474]
            frame False {
            }
            frame True {
              n155 = for {
                tunnel: w1478 -> [w1483] mode=indexing
                shift-right: [w1487] -> w1476
                shift-left: w1474 -> [w1486]
                tunnel: w1477 -> [w1489]
                i -> [w1488]
                n156 = Greater?(x="decimating factor", y=1) -> (0:w1482:bool)
                n157 = call-poly <vilib>:"Decimate (single shot).vi"("averaging"=TRUE, "decimating factor"="decimating factor", "X"=w1483) -> ("Decimated Array"=w1485:dbl[])  [unwired: 7 in, 1 out]
                n158 = Select(t=w1485, s=w1482, f=w1483) -> (s? t:f=w1484:dbl[])
                n159 = for {
                  tunnel: w1484 -> [w1496] mode=indexing
                  shift-right: [w1495] -> w1487
                  shift-left: w1486 -> [w1493]
                  tunnel: w1489 -> [w1498]
                  tunnel: w1488 -> [w1497]
                  tunnel: "decimating factor" -> [w1490]
                  i -> [w1499]
                  n160 = Multiply(x=w1498, y=w1499) -> (x*y=w1492:dbl)
                  n161 = Multiply(x=w1490, y=w1492) -> (x*y=w1491:dbl)
                  n162 = Build Array(w1497, w1491, w1496) -> (w1494:dbl[])
                  n163 = Build Array (concatenate)(w1493, w1494) -> (w1495:dbl[][])
                }
              }
              n164 = call-poly <vilib>:"Write To Spreadsheet File.vi"("format (%.3f)"="%.10f", "2D data"=w1476) -> ()  [unwired: 6 in, 1 out]
            }
          }
          n165 = case shown="True" "Save Coefficients" {
            tunnel: w1451 -> [_ w1471]
            frame False {
            }
            frame True {
              n166 = call-poly <vilib>:"Write To Spreadsheet File.vi"("format (%.3f)"="%.10f", "append to file? (new file:F)"=TRUE, "1D data"=w1471) -> ()  [unwired: 5 in, 1 out]
            }
          }
          n167 = property on="Event-related responses" class="WFGraph (strict)"() -> ("CrsrList"=w1444:T4)  [unwired: 2 in, 2 out]
          n168 = Index Array(array=w1444, index=0) -> (element=w1443:T5)
          n169 = Index Array(array=w1444, index=1) -> (element=w1442:T5)
          n170 = Unbundle By Name(w1443) -> ("Position.X"=w1441:dbl)
          n171 = Unbundle By Name(w1442) -> ("Position.X"=w1440:dbl)
          n172 = Max & Min(x=w1441, y=w1440) -> (max(x,y)=w1439:dbl, min(x,y)=w1438:dbl)
          n173 = case shown="True" "Save Between Cursors" {
            tunnel: w1447 -> [_ w1465]
            tunnel: w1439 -> [_ w1462]
            tunnel: w1438 -> [_ w1461]
            tunnel: w1437 -> [_ w1463]
            frame False {
            }
            frame True {
              n174 = Divide(x=w1461, y=w1463) -> (x/y=w1459:dbl)
              n175 = Divide(x=w1462, y=w1463) -> (x/y=w1460:dbl)
              n176 = Subtract(x=w1460, y=w1459) -> (x-y=w1464:dbl)
              n177 = for {
                tunnel: w1465 -> [w1470] mode=indexing
                tunnel: w1464 -> [w1469]
                tunnel: w1459 -> [w1468]
                tunnel: [w1466] -> w1458 mode=indexing
                n178 = Array Subset(array=w1470, index=w1468, length=w1469) -> (w1467:dbl[])
                n179 = call-poly <vilib>:"Mean.vi"("X"=w1467) -> ("mean"=w1466:dbl)  [unwired: 1 out]
              }
              n180 = call-poly <vilib>:"Write To Spreadsheet File.vi"("format (%.3f)"="%.10f", "append to file? (new file:F)"=TRUE, "1D data"=w1458) -> ()  [unwired: 5 in, 1 out]
            }
          }
        }
        n181 = property on="Event-related responses" class="WFGraph (strict)"("XScale.Multiplier"=w1366) -> ()  [unwired: 2 in, 2 out]
        "Tab Control" <- enum32{"Data Cleaning", "Pupil Analysis"}."Pupil Analysis" ("Tab Control")
      }
    }
    frame #2 {
      n182 = for {
        tunnel: w1555 -> [w1602] mode=indexing
        tunnel: w1554 -> [w1611]
        shift-right: [w1563] -> _
        shift-left: dbl[][] [] -> [w1564]
        i -> [w1582]
        n183 = Initialize Array(0.0 ("element"), 600 ("dimension size"), 800 ("dimension size")) -> (w1579:dbl[][])
        n184 = Spreadsheet String To Array(format string="", spreadsheet string=w1602, array type (2D Dbl)=dbl[][] []) -> (array=w1616:dbl[][])  [unwired: 1 in]
        n185 = Index Array(array=w1616, index (row)=0, index (col)=1 ("disabled index (col)")) -> (element=w1609:dbl)
        n186 = Index Array(array=w1611, index=2) -> (element=w1608:waveform(dbl))
        n187 = Index Array(array=w1611, index=3) -> (element=w1607:waveform(dbl))
        n188 = Unbundle By Name(w1608) -> ("Y"=w1606:dbl[], "dt"=w1569:dbl)
        n189 = Divide(x="Post-Picture Window Length", y=w1569) -> (x/y=w1571:dbl)
        n190 = Divide(x=w1609, y=w1569) -> (x/y=w1604:dbl)
        n191 = Unbundle By Name(w1607) -> ("Y"=w1605:dbl[])
        n192 = for {
          N: w1571 -> [_]
          tunnel: w1606 -> [w1669]
          tunnel: w1605 -> [w1666]
          tunnel: w1604 -> [w1667]
          shift-right: [w1661] -> w1577
          shift-left: w1579 -> [w1664]
          i -> [w1668]
          n193 = Add(x=w1667, y=w1668) -> (x+y=w1665:dbl)
          n194 = Index Array(array=w1669, index=w1665) -> (element=w1663:dbl)
          n195 = Index Array(array=w1666, index=w1665) -> (element=w1662:dbl)
          n196 = Multiply(x=w1662, y=800) -> (x*y=w1660:dbl)
          n197 = Multiply(x=w1663, y=600.0) -> (x*y=w1659:dbl)
          n198 = in-place {
            n199 = in-place-array #1(w1664, w1659, w1660) -> (w1671:dbl)
            n200 = Increment(x=w1671) -> (x+1=w1670:dbl)
            n201 = in-place-array #1(w1670) -> (w1661:dbl[][])  [unwired: 2 out]
          }
        }
        n202 = Array Max & Min(array=w1577) -> (max value=w1588:dbl, min value=w1589:dbl)  [unwired: 2 out]
        n203 = Match Pattern(string=w1602, regular expression="c[^]+\\.bmp") -> (match substring=w1600:string)  [unwired: 1 in, 3 out]
        n204 = Subtract(x=w1588, y=w1589) -> (x-y=w1587:dbl)
        n205 = String To Path(string=w1600) -> (path=w1599:path)
        n206 = Divide(x=256.0, y=w1587) -> (x/y=w1585:dbl)
        n207 = Multiply(x=w1577, y=w1585) -> (x*y=w1584:dbl[][])
        n208 = Strip Path(path=w1599) -> (name=w1597:string)  [unwired: 1 out]
        n209 = call <vilib>:"Search and Replace Pattern.vi"("string"=w1597, "regular expression (\"\")"="\\.bmp" ("regular expression (\"\")"), "replace string (\"\")"=".obt" ("replace string (\"\")")) -> ("result string"=w1593:string)  [unwired: 2 in, 1 out]
        n210 = Build Path(base path="Images Directory", name or relative path=w1597) -> (appended path=w1598:path)
        "Image file" <- w1598
        n211 = call <vilib>:"Flatten Pixmap.vi"("8-bit pixmap"=w1584) -> ("image data"=w1574:T3)  [unwired: 10 in]
        n212 = call <vilib>:"Create Mask.vi"("Mask Color (Black)"=u32 0, "image data"=w1574) -> ("image data"=w1572:T3)  [unwired: 9 in]
        n213 = Build Path(base path="Objects Directory", name or relative path=w1593) -> (appended path=w1591:path)
        "object file" <- w1591
        n214 = call <vilib>:"Read BMP File.vi"("path to BMP file"=w1598) -> ("error out"=w1567:errorcluster, "image data"=w1581:T3)  [unwired: 8 in, 1 out]
        "image data" <- w1581
        n215 = Read from Text File(file (use dialog)=w1591) -> (text=w1590:string, error out=w1568:errorcluster)  [unwired: 3 in, 2 out]
        n216 = call <vilib>:"Draw Flattened Pixmap.vi"("image data"=w1572) -> ("new picture"=w1583:picture)  [unwired: 8 in]
        n217 = Merge Errors(w1567, w1568) -> (w1566:errorcluster)
        n218 = case shown="No Error" w1566 {
          tunnel: [w1620 dbl[] []] -> w1565
          tunnel: w1590 -> [w1619 _]
          tunnel: w1577 -> [w1618 _]
          tunnel: w1583 -> [w1617 _]
          frame No Error {
            n219 = while {
              tunnel: w1618 -> [w1627]
              tunnel: [w1626] -> w1620 mode=indexing
              shift-right: [w1624] -> _
              shift-left: w1617 -> [w1621]
              shift-right: [w1622] -> _
              shift-left: w1619 -> [w1623]
              stop <- w1628 stop-if-true
              n220 = Match Pattern(string=w1623, regular expression="Object[0-9]+=") -> (after substring=w1625:string)  [unwired: 1 in, 3 out]
              n221 = String Subset(string=w1625, length (rest)=1) -> (substring=w1630:string)  [unwired: 1 in]
              n222 = Equal?(x=w1630, y="0") -> (x = y?=w1628:bool)
              n223 = case shown="False" w1628 {
                tunnel: w1625 -> [w1646 w1652]
                tunnel: w1627 -> [w1640 _]
                tunnel: [w1636 0.0 ("Fixations in ROI")] -> w1626
                tunnel: [w1633 w1653] -> w1624
                tunnel: [w1635 w1652] -> w1622
                tunnel: w1621 -> [w1634 w1653]
                frame False {
                  n224 = Match Pattern(string=w1646, regular expression="[0-9]+,") -> (match substring=w1642:string, after substring=w1643:string)  [unwired: 1 in, 2 out]
                  n225 = Decimal String To Number(string=w1642, offset=0) -> (number=w1639:i32)  [unwired: 1 in, 1 out]
                  n226 = for {
                    N: 4 -> [_]
                    shift-right: [w1650] -> w1635
                    shift-left: w1643 -> [w1651]
                    tunnel: [w1648] -> w1638 mode=indexing
                    n227 = Match Pattern(string=w1651, regular expression="[0-9]+") -> (match substring=w1649:string, after substring=w1650:string)  [unwired: 1 in, 2 out]
                    n228 = Decimal String To Number(string=w1649) -> (number=w1648:i32)  [unwired: 2 in, 1 out]
                  }
                  n229 = Array To Cluster(array=w1638) -> (cluster=w1637:T6)
                  n230 = call "FixationInROI.vi"("ROI rect"=w1637, "ROI Type"=w1639, "old picture"=w1634, "Fixations Array"=w1640) -> ("Fixations in ROI"=w1636:dbl, "new picture"=w1633:picture)
                  "2D Picture" <- w1633
                }
                frame True {
                }
              }
            }
          }
          frame Error {
          }
        }
        n231 = call <vilib>:"Draw Flattened Pixmap.vi"("image data"=w1581) -> ("new picture"=→"2D Picture 2":picture)  [unwired: 8 in]
        n232 = while {
          tunnel: w1565 -> [_]
          stop <- "next picture" stop-if-true
        }
        n233 = Build Array (concatenate)(w1564, w1565) -> (w1563:dbl[][])
        "Fixations in ROIs" <- w1563
        "Image Number" <- w1582
      }
      n234 = Index Array(array=w1554, index=2) -> (element=w1562:waveform(dbl))
      n235 = Index Array(array=w1554, index=3) -> (element=w1559:waveform(dbl))
      n236 = Unbundle By Name(w1562) -> ("Y"=w1557:dbl[])  [unwired: 1 out]
      n237 = Unbundle By Name(w1559) -> ("Y"=w1558:dbl[])  [unwired: 1 out]
      n238 = local write "Tab Control"(T1."Eye Tracking Anlysis" ("Tab Control")) -> ()
      n239 = Array Size(array=w1557) -> (size(s)=w1556:i32)
      n240 = for {
        N: w1556 -> [w1683]
        tunnel: w1557 -> [w1686]
        tunnel: w1558 -> [w1682]
        tunnel: [w1672] -> _ mode=indexing
        n241 = Index Array(array=w1686, index=w1683) -> (element=w1680:dbl)
        n242 = Index Array(array=w1682, index=w1683) -> (element=w1676:dbl)
        n243 = Decrement(x=w1683) -> (x-1=w1685:i32)
        n244 = Decrement(x=w1683) -> (x-1=w1684:i32)
        n245 = Index Array(array=w1686, index=w1685) -> (element=w1681:dbl)
        n246 = Index Array(array=w1682, index=w1684) -> (element=w1677:dbl)
        n247 = Subtract(x=w1680, y=w1681) -> (x-y=w1679:dbl)
        n248 = Subtract(x=w1676, y=w1677) -> (x-y=w1678:dbl)
        n249 = Square(x=w1679) -> (x^2=w1675:dbl)
        n250 = Square(x=w1678) -> (x^2=w1674:dbl)
        n251 = Add(x=w1675, y=w1674) -> (x+y=w1673:dbl)
        n252 = Square Root(x=w1673) -> (sqrt(x)=w1672:dbl)
      }
    }
  }
